vi "display Log.vi"(8 "error in (no error)":errorcluster) -> (0 "error out":errorcluster, 3 "function return":string)   [LabVIEW 2019, in "libConvectionDiffusionWrapper.lvlib"]
doc: "char* displayLog();"
uses:
  libConvectionDiffusionWrapper.lvlib
  libConvectionDiffusionWrapper.so
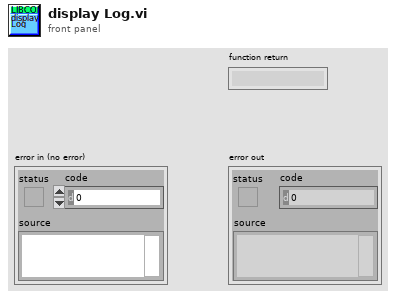
[diagram p1: front panel]
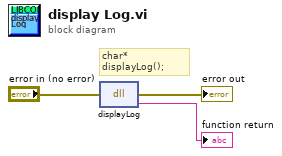
[diagram p0: block diagram]
diagram:
  # "char* displayLog();"
  n1 = dll-call lib="home/paul/Schreibtisch/Convection_diffusion/LabView/lib/libConvectionDiffusionWrapper.*" fn="displayLog"(error in="error in (no error)") -> (error out=→"error out":errorcluster, →"function return":string)  [unwired: 2 in, 1 out]
